vi "IntakeSystem.vi"() -> ()   [LabVIEW 2025]
panel:
  out "IntakeSystem/IntakeAngleTarget":dbl caption="Position Dmd Deg" format="%12.1f"
  out "IntakeSystem/IntakeMotorRPM":dbl caption="Intake RPM" format="%12.1f"
  out "IntakeSystem/IntakeMotorOut":dbl caption="Intake Motor Dmd" format="%11.2f"
  out "Intake/Position":dbl caption="Position Act Deg" format="%12.1f"
  out "IntakeSystem/IntakeLimitIsPressed":bool caption="LowLimitSwitch"
  out "IntakeSystem/IntakeIsExtended":bool caption="Extended"
  # "INTAKE"
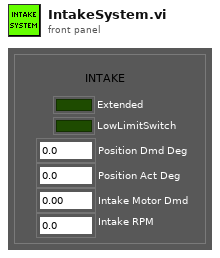
[diagram p1: front panel]
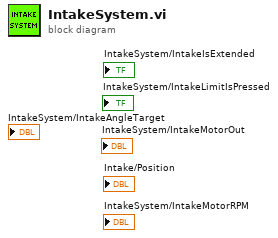
[diagram p0: block diagram]
diagram:
